vi "CPP_Aeroprobe_dT-Unified.vi"() -> (5 "Plug in titles":string[](array[string]), 7 "Plug in values":string[](array[string]))   [LabVIEW 2013]
uses:
  Plug in sub vis/CPP_Aeroprobe/SanityCluster.ctl
  <vilib>/Analysis/baseanly.llb/Mean (DBL).vi
  Globals/Meas_global.vi
  Globals/Trav_pos_global.vi
  <vilib>/Analysis/NI_AALBase.lvlib
panel:
  in  "Mode":enum32{"Measure", "Take Zeroes"}(radio)
  in  "RunManually?":bool
  in  "MeanOrFull":bool
  in  "Graphs":bool
  in  "Downsampler":i32=80
  in  "Calibration Folder Path":path=path "M:/Preferences/Rig_Setups/All_Rigs/Calibrations/5HoleProbeRegrid"
  in  "Correction File Path":path=path "M:/Preferences/Rig_Setups/All_Rigs/TubingCompensation/5HPTubingCorrection12066.xls"
  # "!! 5-hole 1-5 must be connected to Channels 1-5 !!"
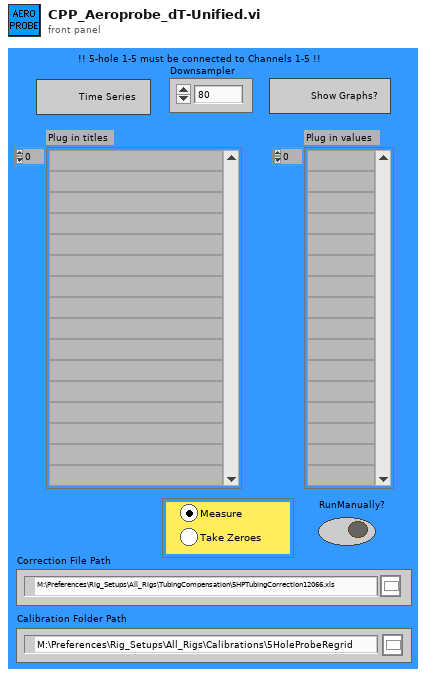
[diagram p1: front panel]
types:
  T1 = typedef "SanityCluster.ctl" = cluster{"PressureErrors":bool[][], "Plug in titles":string[]}
  T2 = typedef "Post_Process.ctl" = enum16{"Take New Data", "Post Process Raw Data File"}
  T3 = typedef "Traverse_cluster.ctl" = cluster{"Start X":dbl, "Start Y":dbl, "Start Z":dbl, "End X":dbl, "End Y":dbl, "End Z":dbl, "No. of pts.":i32, "Spacing":T4, "Filename":path, "Tunnel Speed":dbl, "Averaging time (min)":dbl, "Extra Commands":string, "Specific Arguments":string, "Emission Rate (l/min)":dbl, "Trace Gas Concentration (%)":dbl, "Density Ratio":string, "Comments":string, "Row No":i32, "Row Type Selector":T5, "Completion time":string, "Row Duration (mins)":dbl, "No. of Valid pts.":i32, "Meas Setup File":string}
  T4 = typedef "Spacing.ctl" = enum16{"Linear", "Log", "Gauss", "Specified", "N/A"}
  T5 = typedef "Multi_run_mode.ctl" = enum16{"Move Traverse Only", "Set Tunnel Speed Only", "Set Source Only", "Set Measurement Conditions", "Single Measurement", "Vertical Profile", "Lateral Profile", "Longitudinal Profile", "Explore Volume", "Multi-Axis Profile", "Auto Calibrate", "Meas Fast FID Bkgnd", "Check Beam Power", "Scanning Valve Measurement", "Run VI Named:", "Set ADAM Ch", "Wait (minutes)", "Send Message", "Synchronize With:", "Fall Back to this Row", "Turn Off Row Repeating", "Blank Row", "Traverse 3D Volume"}
  T6 = typedef "Analysis_info_cluster.ctl" = cluster{"Colour":u32, "Inst type":T7, "Inst name":string, "Symbol":string, "Code name":string, "Extra Info":string, "Inst Array":T8, "Extra Titles":string[], "Extra Values":string[], "U":dbl, "u^2":dbl, "u^3":dbl, "u^4":dbl, "Skew_u":dbl, "Kurt_u":dbl, "Sd Error in Mean":dbl, "% u'/U":dbl, "X":dbl, "Y":dbl, "Z":dbl, "Timescale integral to 25%":dbl, "Sd Error in Variance":dbl, "Calib File":path, "Calib Constants":dbl[], "Output Position":bool, "Full Stats":bool, "Av Sampling Rate":dbl, "Av No of Samples":dbl, "Total Meas Time (s)":dbl, "ADAM Ch Name":string}
  T7 = typedef "Inst_type.ctl" = enum16{"Propeller anemometer", "Raw voltage", "Pressure Transducer", "Pitot-static tube", "Preston tube", "Hot wire", "Cross wire 1", "Cross wire 2", "Generic Linear", "Generic Polynomial", "Generic BackPoly", "Fast FID", "Thermocouple", "Cold wire", "Pulsed Wire", "LDA Vel", "LDA Tran time", "LDA Arr time"}
  T8 = typedef "Instrument_Array.ctl" = enum16{"PWA", "LDA", "Analogue"}
  T9 = cluster{"Analysis Info cluster[0]":T6, "Analysis Info cluster[1]":T6, "Analysis Info cluster[2]":T6, "Analysis Info cluster[3]":T6, "Analysis Info cluster[4]":T6, "Analysis Info cluster[5]":T6, "Analysis Info cluster[6]":T6}
  T10 = typedef "Time_Trace_Cluster.ctl" = cluster{"Weighting":dbl[], "Time (s)":dbl[], "Voltage":dbl[], "Eng Values":dbl[]}
  T11 = typedef "GoodArray.ctl" = bool[]
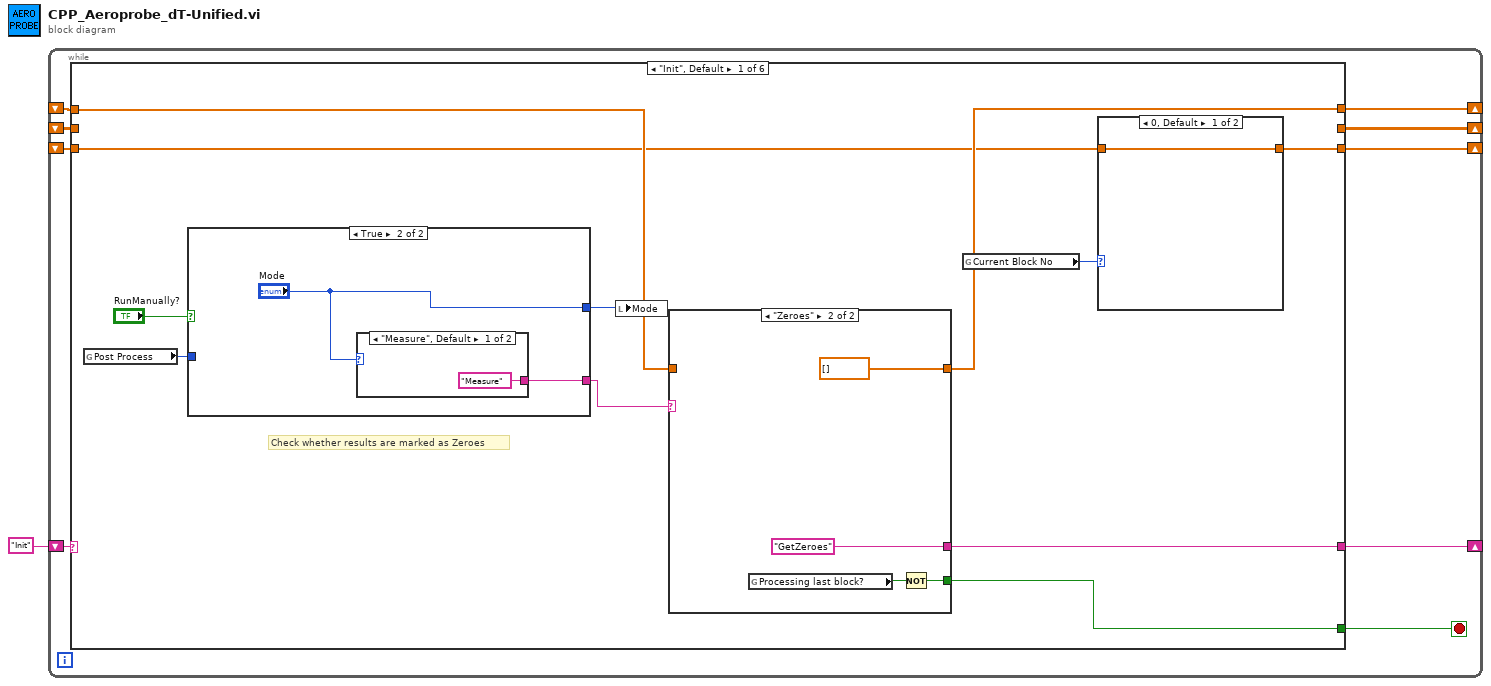
[diagram p0: block diagram]
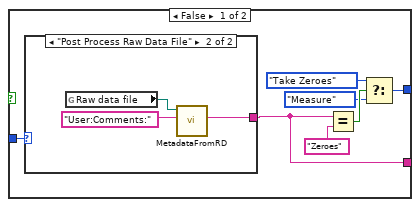
[diagram p2: hidden frame]
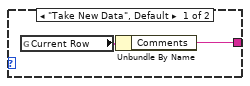
[diagram p3: hidden frame]
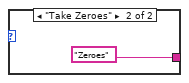
[diagram p4: hidden frame]
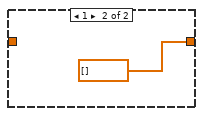
[diagram p5: hidden frame]
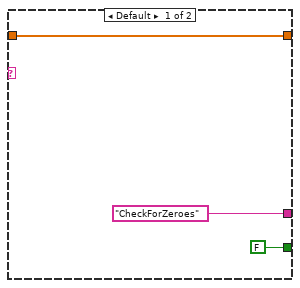
[diagram p6: hidden frame]
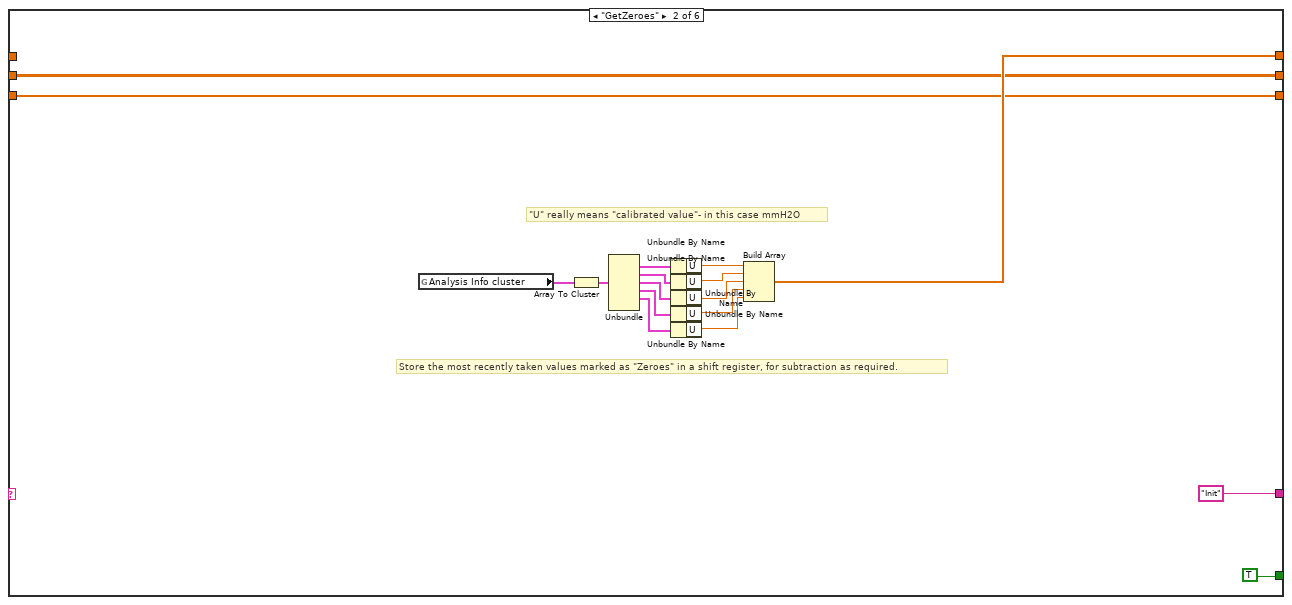
[diagram p7: hidden frame]
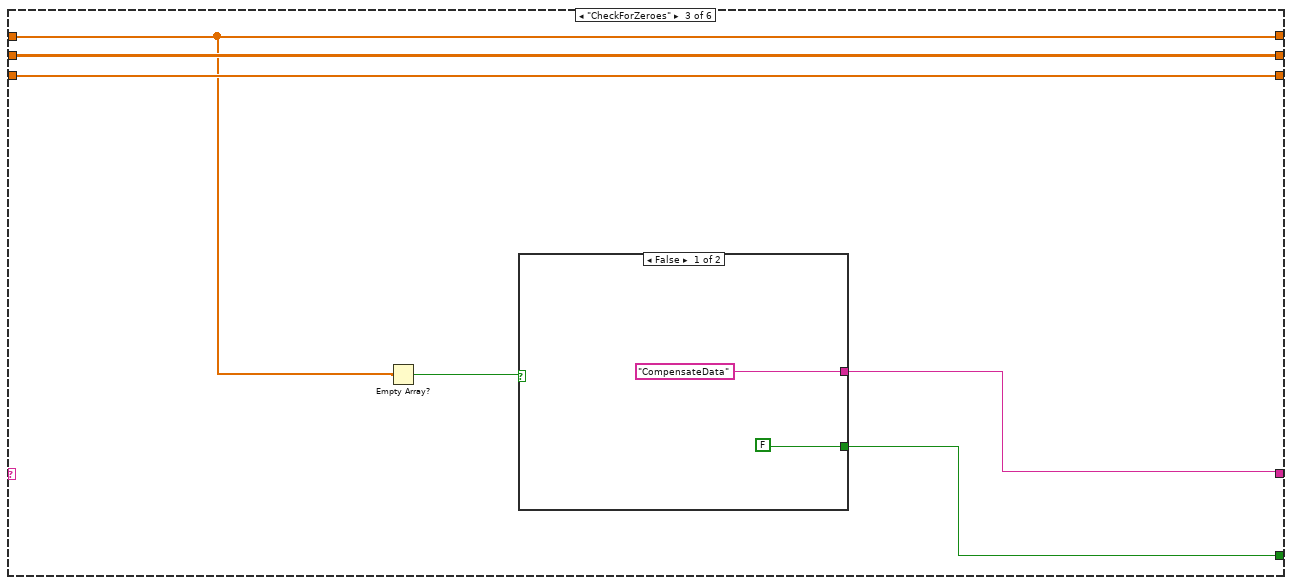
[diagram p8: hidden frame]
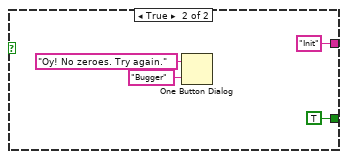
[diagram p9: hidden frame]
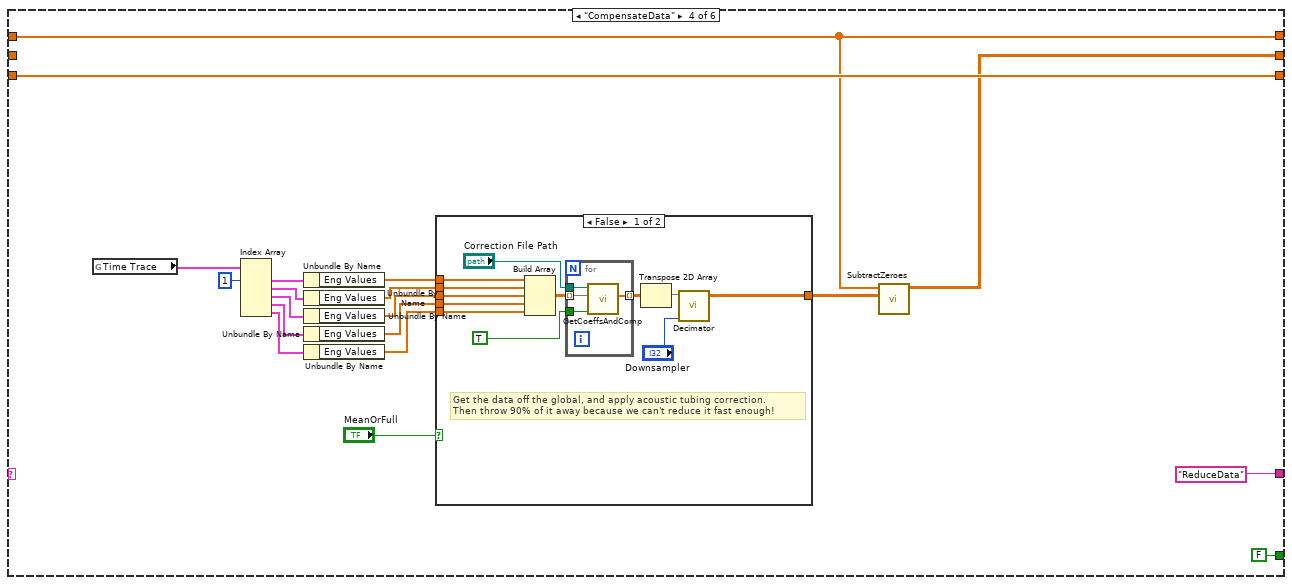
[diagram p10: hidden frame]
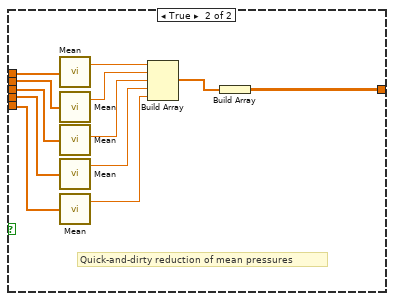
[diagram p11: hidden frame]
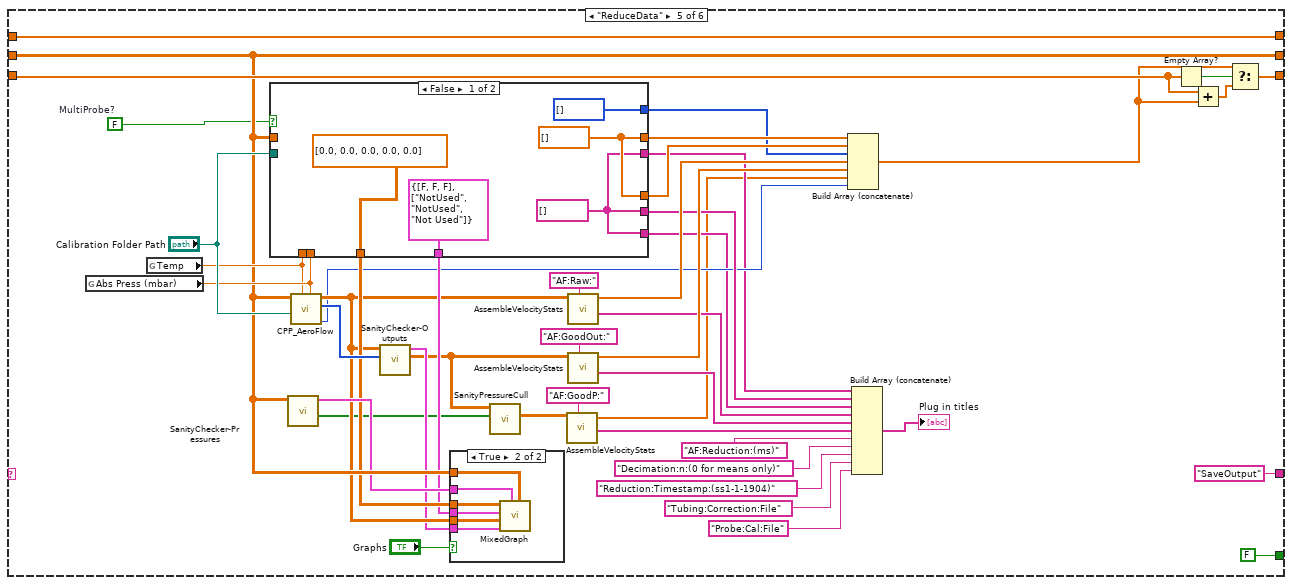
[diagram p12: hidden frame]
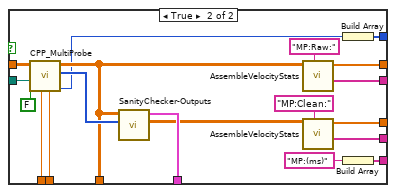
[diagram p13: hidden frame]
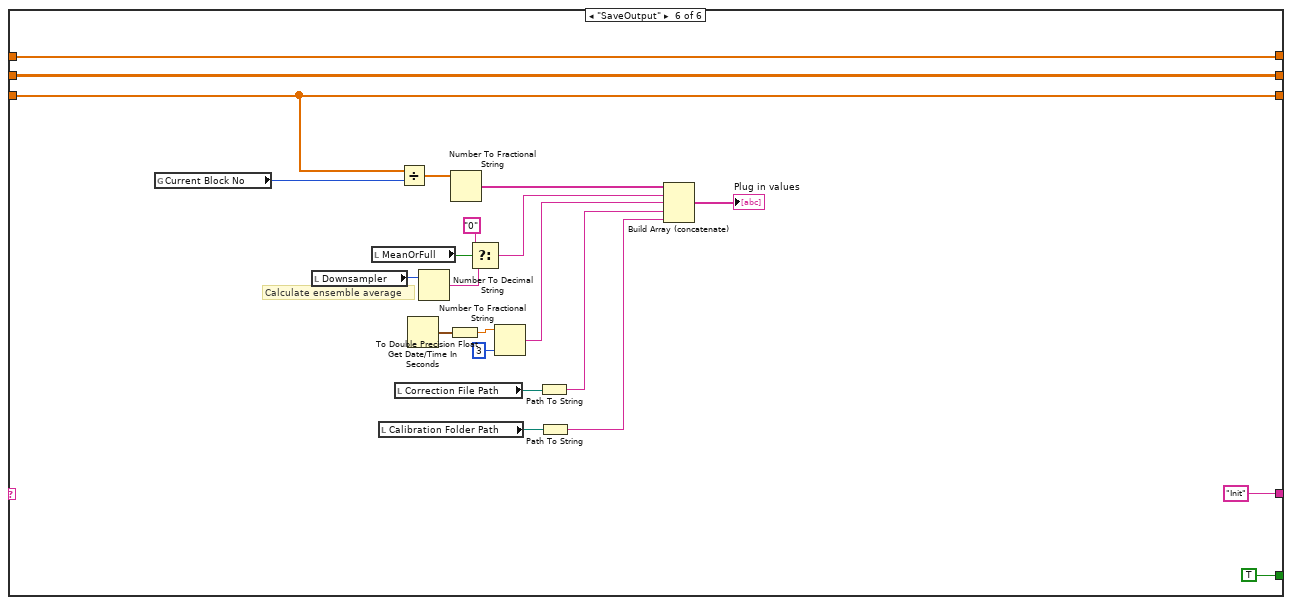
[diagram p15: hidden frame]
diagram:
  n1 = while {
    shift-right: [w9] -> _
    shift-left: "Init" -> [w10]
    shift-right: [w8] -> _
    shift-left: _ -> [w7]
    shift-right: [w6] -> _
    shift-left: _ -> [w5]
    shift-right: [w3] -> _
    shift-left: _ -> [w2]
    stop <- w4 stop-if-true
    n2 = case shown="\"Init\", Default" w10 {
      tunnel: [w21 "Init" w68 "ReduceData" "SaveOutput" "Init"] -> w9
      tunnel: [w18 w50 w65 w80 w166 w219] -> w8
      tunnel: w7 -> [w19 _ w65 w80 w166 w219]
      tunnel: [w17 w48 w69 w94 w161 w213] -> w6
      tunnel: w5 -> [w16 w48 w69 w94 w164 w213]
      tunnel: [w20 TRUE w67 FALSE FALSE TRUE] -> w4
      tunnel: [_ w47 w66 w77 w153 w215] -> w3
      tunnel: w2 -> [_ w47 w66 _ w153 w215]
      frame "Init", Default {
        # "Check whether results are marked as Zeroes"
        n3 = global read "Meas_global.vi" "Post Process"() -> (w12:T2)
        n4 = case shown="True" "RunManually?" {
          tunnel: [w28 "Mode"] -> w13
          tunnel: w12 -> [w23 _]
          tunnel: [w22 w34] -> w11
          frame False {
            n5 = case shown="\"Post Process Raw Data File\"" w23 {
              tunnel: [w29 w31] -> w22
              frame "Take New Data", Default {
                n6 = global read "Trav_pos_global.vi" "Current Row"() -> (w30:T3)
                n7 = Unbundle By Name(w30) -> ("Comments"=w29:string)
              }
              frame "Post Process Raw Data File" {
                n8 = global read "Meas_global.vi" "Raw data file"() -> (w33:path)
                n9 = call "MetadataFromRD.vi"("ChannelName"="User:Comments:", "Raw data file"=w33) -> ("ValueString"=w31:string)  [unwired: 8 in, 1 out]
              }
            }
            n10 = Equal?(x=w22, y="Zeroes") -> (x = y?=w26:bool)
            n11 = Select(t=enum32{"Measure", "Take Zeroes"}."Take Zeroes" ("Mode"), s=w26, f=enum32{"Measure", "Take Zeroes"}."Measure" ("Mode")) -> (s? t:f=w28:enum32{"Measure", "Take Zeroes"})
          }
          frame True {
            n12 = case shown="\"Measure\", Default" "Mode" {
              tunnel: ["Measure" ("y") "Zeroes" ("y")] -> w34
              frame "Measure", Default {
              }
              frame "Take Zeroes" {
              }
            }
          }
        }
        n13 = local write "Mode"(w13) -> ()
        n14 = case shown="\"Zeroes\"" w11 {
          tunnel: ["CheckForZeroes" "GetZeroes"] -> w21
          tunnel: [FALSE w45] -> w20
          tunnel: w19 -> [w40 _]
          tunnel: [w40 dbl[] [] ("t")] -> w18
          frame Default {
          }
          frame "Zeroes" {
            n15 = global read "Meas_global.vi" "Processing last block?"() -> (w44:bool)
            n16 = Not(x=w44) -> (.not. x?=w45:bool)
          }
        }
        n17 = global read "Meas_global.vi" "Current Block No"() -> (w15:i32)
        n18 = case shown="0, Default" w15 {
          tunnel: [w38 dbl[] [] ("t")] -> w17
          tunnel: w16 -> [w38 _]
          frame 0, Default {
          }
          frame 1 {
          }
        }
      }
      frame "GetZeroes" {
        # "Store the most recently taken values marked as \"Zeroes\" in a shift register, for subtraction as required."
        # "\"U\" really means \"calibrated value\"- in this case mmH2O"
        n19 = global read "Meas_global.vi" "Analysis Info cluster"() -> (w52:T6[])
        n20 = Array To Cluster(array=w52) -> (cluster=w58:T9)
        n21 = Unbundle(w58) -> ("Analysis Info cluster[1]"=w59:T6, "Analysis Info cluster[2]"=w60:T6, "Analysis Info cluster[3]"=w61:T6, "Analysis Info cluster[4]"=w62:T6, "Analysis Info cluster[5]"=w63:T6)  [unwired: 2 out]
        n22 = Unbundle By Name(w59) -> ("U"=w57:dbl)
        n23 = Unbundle By Name(w60) -> ("U"=w56:dbl)
        n24 = Unbundle By Name(w61) -> ("U"=w55:dbl)
        n25 = Unbundle By Name(w62) -> ("U"=w54:dbl)
        n26 = Unbundle By Name(w63) -> ("U"=w53:dbl)
        n27 = Build Array(w57, w56, w55, w54, w53) -> (w50:dbl[])
      }
      frame "CheckForZeroes" {
        n28 = Empty Array?(array=w65) -> (empty?=w64:bool)
        n29 = case shown="False" w64 {
          tunnel: ["CompensateData" "Init"] -> w68
          tunnel: [FALSE TRUE] -> w67
          frame False {
          }
          frame True {
            n30 = One Button Dialog(message="Oy! No zeroes. Try again.", button name ("OK")="Bugger") -> ()  [unwired: 1 out]
          }
        }
      }
      frame "CompensateData" {
        n31 = global read "Meas_global.vi" "Time Trace"() -> (w84:T10[])
        n32 = Index Array(array=w84, index #1=1 ("index")) -> (element #1=w83:T10, element #2=w92:T10, element #3=w91:T10, element #4=w90:T10, element #5=w89:T10)  [unwired: 4 in]
        n33 = Unbundle By Name(w83) -> ("Eng Values"=w82:dbl[])
        n34 = Unbundle By Name(w92) -> ("Eng Values"=w88:dbl[])
        n35 = Unbundle By Name(w91) -> ("Eng Values"=w87:dbl[])
        n36 = Unbundle By Name(w90) -> ("Eng Values"=w86:dbl[])
        n37 = Unbundle By Name(w89) -> ("Eng Values"=w85:dbl[])
        n38 = case shown="False" "MeanOrFull" {
          tunnel: w88 -> [w106 w121]
          tunnel: w87 -> [w105 w120]
          tunnel: w86 -> [w104 w119]
          tunnel: w85 -> [w103 w118]
          tunnel: w82 -> [w102 w122]
          tunnel: [w95 w111] -> w81
          frame False {
            # "Get the data off the global, and apply acoustic tubing correction. \nThen throw 90% of it away because we can't reduce it fast enough!"
            n39 = Build Array(w102, w106, w105, w104, w103) -> (w101:dbl[][])
            n40 = for {
              tunnel: w101 -> [w110] mode=indexing
              tunnel: [w109] -> w98 mode=indexing
              tunnel: TRUE ("Apply Phase Correction?") -> [w108]
              tunnel: "Correction File Path" -> [w107]
              n41 = call "GetCoeffsAndComp.vi"("Apply Phase Correction?"=w108, "mutedData"=w110, "TubingCorrectionFile"=w107) -> ("boostedData"=w109:dbl[])  [unwired: 8 in]
            }
            n42 = Transpose 2D Array(2D array=w98) -> (transposed array=w97:dbl[][])
            n43 = call "Decimator.vi"("Decimator"="Downsampler", "Array In"=w97) -> ("DecimatedArrayOut"=w95:dbl[][])  [unwired: 9 in]
          }
          frame True {
            # "Quick-and-dirty reduction of mean pressures"
            n44 = call-poly <vilib>:"Mean.vi"("X"=w122) -> ("mean"=w117:dbl)  [unwired: 1 out]
            n45 = call-poly <vilib>:"Mean.vi"("X"=w121) -> ("mean"=w116:dbl)  [unwired: 1 out]
            n46 = call-poly <vilib>:"Mean.vi"("X"=w120) -> ("mean"=w115:dbl)  [unwired: 1 out]
            n47 = call-poly <vilib>:"Mean.vi"("X"=w119) -> ("mean"=w114:dbl)  [unwired: 1 out]
            n48 = call-poly <vilib>:"Mean.vi"("X"=w118) -> ("mean"=w113:dbl)  [unwired: 1 out]
            n49 = Build Array(w117, w116, w115, w114, w113) -> (w112:dbl[])
            n50 = Build Array(w112) -> (w111:dbl[][])
          }
        }
        n51 = call "SubtractZeroes.vi"("RawPressure"=w81, "Zeroes"=w80) -> ("ZeroedPressure"=w77:dbl[][])  [unwired: 9 in]
      }
      frame "ReduceData" {
        w134 = FALSE  # MultiProbe?
        n52 = global read "Meas_global.vi" "Abs Press (mbar)"() -> (w158:dbl)
        n53 = global read "Meas_global.vi" "Temp"() -> (w157:dbl)
        n54 = case shown="False" w134 {
          tunnel: [w172 w191] -> w160
          tunnel: "Calibration Folder Path" -> [_ w190]
          tunnel: w158 -> [_ w189]
          tunnel: w157 -> [_ w188]
          tunnel: w153 -> [_ w184]
          tunnel: [dbl[][] [[0.0, 0.0, 0.0, 0.0, 0.0]] ("RawVmagUVWCone") w183] -> w151
          tunnel: [T1 {"PressureErrors"=[[FALSE, FALSE, FALSE]], "Plug in titles"=["NotUsed", "NotUsed", "Not Used"]} ("OutputErrors") w182] -> w150
          tunnel: [w172 w179] -> w145
          tunnel: [w171 w178] -> w142
          tunnel: [u32[] [] w174] -> w137
          tunnel: [w171 w173] -> w136
          tunnel: [w171 w175] -> w135
          frame False {
            w171 = string[] [] ("Plug in titles")
            w172 = dbl[] [] ("StatsArray")
          }
          frame True {
            n55 = call "CPP_MultiProbe.vi"("Pressure (mBar)"=w189, "Temperature (C)"=w188, "Old5HoleProbe?"=FALSE, "Calibration Folder Path"=w190, "ZeroedPressures (mmH2O)"=w184) -> ("Time (ms)"=w177:u32, "ReductionCode"=w185:i32[], "RawVmagUVWCone"=w183:dbl[][])  [unwired: 1 in, 1 out]
            n56 = call "SanityChecker-Outputs.vi"("ReductionCode"=w185, "RawVmagUVWCone"=w183) -> ("SanitisedVmagUVWCone"=w181:dbl[][], "OutputErrors"=w182:T1)  [unwired: 7 in, 1 out]
            n57 = call "AssembleVelocityStats.vi"("TitlePrefix"="MP:Raw:", "VmagUVWCone"=w183) -> ("Plug in titles"=w175:string[], "StatsArray"=w191:dbl[])  [unwired: 8 in]
            n58 = call "AssembleVelocityStats.vi"("TitlePrefix"="MP:Clean:", "VmagUVWCone"=w181) -> ("Plug in titles"=w178:string[], "StatsArray"=w179:dbl[])  [unwired: 8 in]
            n59 = Build Array(w177) -> (w174:u32[])
            n60 = Build Array("MP:(ms)") -> (w173:string[])
          }
        }
        n61 = call "SanityChecker-Pressures.vi"("ZeroedPressures"=w153) -> ("GoodPressures"=w130:T11, "Sanity"=w152:T1)  [unwired: 9 in]
        n62 = call "CPP_AeroFlow.vi"("Pressure (mBar)"=w158, "Temperature (C)"=w157, "Calibration Folder Path"="Calibration Folder Path", "ZeroedPressures (mmH2O)"=w153) -> ("Time(ms)"=w138:u32, "ReductionCode"=w155:i32[], "RawVmagUVWCone"=w149:dbl[][])  [unwired: 2 in, 1 out]
        n63 = call "SanityChecker-Outputs.vi"("ReductionCode"=w155, "RawVmagUVWCone"=w149) -> ("SanitisedVmagUVWCone"=w131:dbl[][], "OutputErrors"=w148:T1)  [unwired: 7 in, 1 out]
        n64 = case shown="True" "Graphs" {
          tunnel: w153 -> [_ w197]
          tunnel: w152 -> [_ w196]
          tunnel: w151 -> [_ w195]
          tunnel: w150 -> [_ w194]
          tunnel: w149 -> [_ w193]
          tunnel: w148 -> [_ w192]
          frame False {
          }
          frame True {
            n65 = call "MixedGraph.vi"("ZeroedPressure"=w197, "PressureSanity"=w196, "OutputErrors2"=w192, "RawVmagUVWCone2"=w193, "OutputErrors1"=w194, "RawVmagUVWCone1"=w195) -> ()  [unwired: 6 in]
          }
        }
        n66 = call "SanityPressureCull.vi"("GoodPressures"=w130, "VmagUVWCone"=w131) -> ("SanitisedVmagUVWCone"=w132:dbl[][])  [unwired: 9 in]
        n67 = call "AssembleVelocityStats.vi"("TitlePrefix"="AF:GoodP:", "VmagUVWCone"=w132) -> ("Plug in titles"=w129:string[], "StatsArray"=w127:dbl[])  [unwired: 8 in]
        n68 = call "AssembleVelocityStats.vi"("TitlePrefix"="AF:Raw:", "VmagUVWCone"=w149) -> ("Plug in titles"=w141:string[], "StatsArray"=w144:dbl[])  [unwired: 8 in]
        n69 = call "AssembleVelocityStats.vi"("TitlePrefix"="AF:GoodOut:", "VmagUVWCone"=w131) -> ("Plug in titles"=w140:string[], "StatsArray"=w143:dbl[])  [unwired: 8 in]
        n70 = Build Array (concatenate)(w160, w145, w137, w144, w143, w127, w138) -> (w146:dbl[])
        n71 = Build Array (concatenate)(w135, w142, w136, w141, w140, w129, "AF:Reduction:(ms)", "Decimation:n:(0 for means only)" ("element"), "Reduction:Timestamp:(ss1-1-1904)" ("element"), "Tubing:Correction:File" ("element"), "Probe:Cal:File" ("element")) -> (→"Plug in titles":string[])
        n72 = Empty Array?(array=w164) -> (empty?=w163:bool)
        n73 = Add(x=w164, y=w146) -> (x+y=w162:dbl[])
        n74 = Select(t=w146, s=w163, f=w162) -> (s? t:f=w161:dbl[])
      }
      frame "SaveOutput" {
        # "Calculate ensemble average"
        n75 = global read "Meas_global.vi" "Current Block No"() -> (w216:i32)
        n76 = local read "Downsampler"() -> (w212:i32)
        n77 = local read "MeanOrFull"() -> (w211:bool)
        n78 = local read "Calibration Folder Path"() -> (w200:path)
        n79 = local read "Correction File Path"() -> (w202:path)
        n80 = Divide(x=w213, y=w216) -> (x/y=w214:dbl[])
        n81 = Get Date/Time In Seconds() -> (seconds since 1Jan1904=w208:timestamp)
        n82 = Number To Decimal String(number=w212) -> (decimal integer string=w210:string)  [unwired: 1 in]
        n83 = To Double Precision Float(number=w208) -> (double precision float=w207:dbl)
        n84 = Number To Fractional String(number=w214) -> (F-format string=w203:string[])  [unwired: 3 in]
        n85 = Select(t="0", s=w211, f=w210) -> (s? t:f=w206:string)
        n86 = Number To Fractional String(number=w207, precision (6)=i16 3) -> (F-format string=w205:string)  [unwired: 2 in]
        n87 = Path To String(path=w202) -> (string=w201:string)
        n88 = Path To String(path=w200) -> (string=w199:string)
        n89 = Build Array (concatenate)(w203, w206, w205, w201, w199) -> (→"Plug in values":string[])
      }
    }
  }
